vi "2108cdc.vi"() -> ()   [LabVIEW 2019]
doc: "This example performs writes and reads on a serial port, as directed by the user. You can press the Write and Read buttons, and change the Read Count, while the example is running.\n\nThe parameters set for the serial port must match the parameters of the connected instrument or device. In this example, the Read Count parameter specifies the number of bytes that the serial port reads. If there were more bytes at the port than the specified number, those bytes would not be read. If there were less bytes at the port than the specified number, you would receive a timeout error.\n\nThis example expands upon the flow control options for XON and XOFF, allowing the user to choose those control characters. Also, the user can enable or disable a termination character. Some devices require a termination character in order to identify the end of command strings. Some devices send a termination character to signify the end of data to be read. This example shows how you can end the Read operation once a termination character is detected in the buffer and/or append a termination character at the end of the Write data."
uses:
  <vilib>/Instr/_visa.llb/VISA Configure Serial Port (Instr).vi
panel:
  in  "Command List":string="stop\neol 1\nencode 1\nslist 0 0\nslist 1 1\nsrate 6000\ndec 500\ndeca 3\nnop\nstart\n"
  in  "Stop":bool
  out "Response":string=" 0.000, 0.000\n 0.000, 0.000\n 0.000, 0.000\n 0.000, 0.000\n 0.000, 0.000\n 0.000, 0.001\n 0.000, 0.001\n 0.000, 0.001\n 0.000, 0.001\n 0.000, 0.001\n 0.000, 0.000\n 0.000, 0.000\n 0.000, 0.000\n 0.000, 0.000\n 0.000, 0.000\n 0.000, 0.001\n 0.000, 0.000\n 0.000, 0.000\n 0.000, 0.000\n 0.000, 0.000\n 0.000, 0.000\n 0.000, 0.001\n 0.000, 0.001\n 0.000, 0.001\n 0.000, 0.000\n 0.000, 0.000\n 0.000, 0.000\n 0.000, 0.000\n 0.000, 0.000\n 0.000, 0.000\n 0.000, 0.000\n 0.000, 0.000\n 0.000, 0.000\n 0.000, 0.000\n 0.000, 0.000\n 0.000, 0.000\n 0.000, 0.000\n 0.000, 0.001\n 0.000, 0.001\n 0.000, 0.000\n 0.000, 0.000\n 0.000, 0.000\n 0.000, 0.001\n 0.000, 0.000\n 0.000, 0.000\n 0.000, 0.001\n 0.000, 0.000\n 0.000, 0.000\n 0.000, 0.000\n 0.000, 0.000\n 0.000, 0.001\n 0.000, 0.000\n 0.000, 0.000\n 0.000, 0.001\n 0.000, 0.000\n 0.000, 0.000\n 0.000, 0.000\n 0.000, 0.000\n 0.000, 0.000\n 0.000, 0.001\n 0.000, 0.000\n 0.000, 0.000\n 0.000, 0.000\n 0.000, 0.000\n 0.000, 0.001\n 0.000, 0.000\n 0.000, 0.000\n 0.000, 0.000\n 0.000, 0.000\n 0.000, 0.000\n 0.000, 0.000\n 0.000, 0.000\n 0.000, 0.000\n 0.000, 0.000\n 0.000, 0.000\n 0.000, 0.000\n"
  in  "2108 CDC Virtual COM":refnum<visa-resource-name>="COM11"
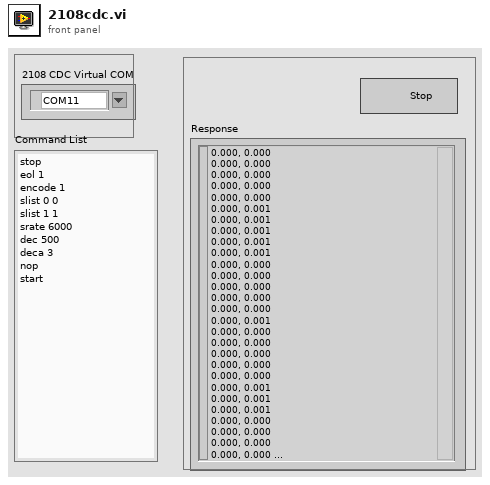
[diagram p1: front panel]
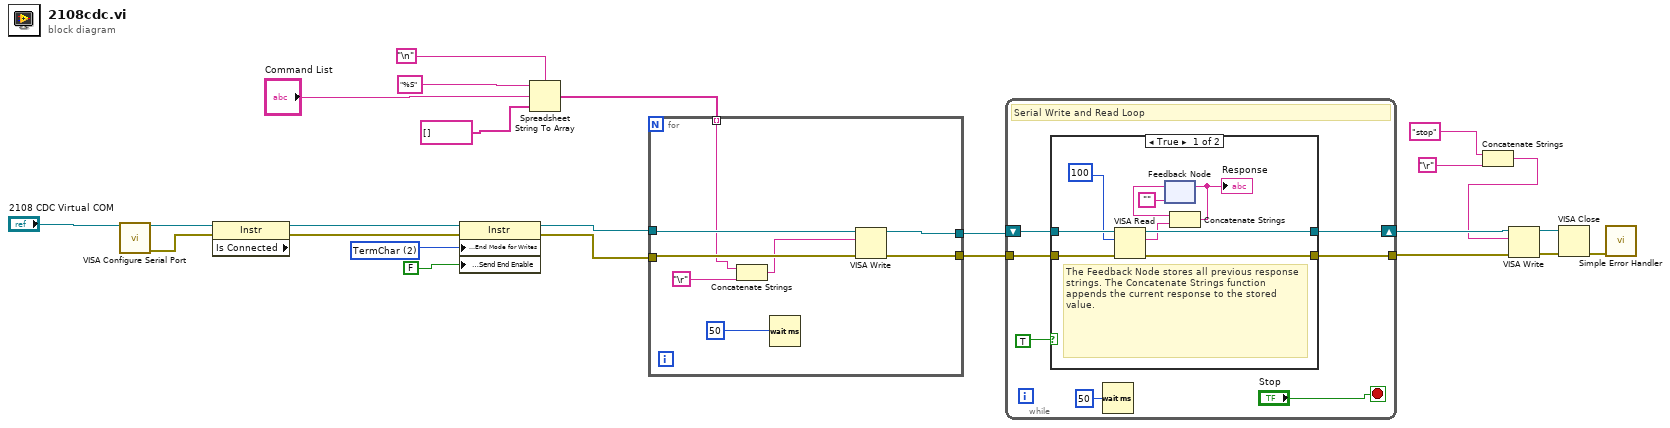
[diagram p0: block diagram]
diagram:
  w21 = u16 2 items=["None", "LastBit", "TermChar", "Break"] ("Serial Settings:Serial End Mode for Writes")
  n1 = call-poly "VISA Configure Serial Port"("VISA resource name"="2108 CDC Virtual COM") -> ("VISA resource name out"=w22:refnum<visa-resource-name>, "error out"=w24:errorcluster)  [unwired: 9 in, 4 out]
  n2 = property class="Instr" props=["Is Connected"](reference=w22, error in=w24) -> (reference out=w19:refnum<visa-resource-name>, error out=w18:errorcluster)  [unwired: 1 out]
  n3 = property class="Instr"(reference=w19, error in=w18, "Serial Settings:End Mode for Writes"=w21, "Message Based Settings:Send End Enable"=FALSE) -> (reference out=w1:refnum<visa-resource-name>, error out=w2:errorcluster)
  n4 = Spreadsheet String To Array(delimiter (Tab)="\n", format string="%S", spreadsheet string="Command List", array type (2D Dbl)=string[] []) -> (array=w14:string[])
  n5 = for {
    tunnel: w14 -> [w29] mode=indexing
    tunnel: w1 -> [w32]
    tunnel: w2 -> [w31]
    tunnel: [w26] -> w4
    tunnel: [w25] -> w3
    n6 = Concatenate Strings(w29, "\r") -> (w27:string)
    n7 = Wait (ms)(milliseconds to wait=u32 50) -> ()  [unwired: 1 out]
    n8 = VISA Write(VISA resource name=w32, write buffer=w27, error in (no error)=w31) -> (VISA resource name out=w26:refnum<visa-resource-name>, error out=w25:errorcluster)  [unwired: 1 out]
  }
  n9 = while {
    shift-right: [w39] -> w11
    shift-left: w4 -> [w35]
    tunnel: w3 -> [w34]
    tunnel: [w37] -> w8
    stop <- "Stop" stop-if-true
    # "Serial Write and Read Loop"
    n10 = case shown="True" TRUE {
      tunnel: [w46 w50] -> w39
      tunnel: w35 -> [w48 w50]
      tunnel: w34 -> [w47 w49]
      tunnel: [w45 w49] -> w37
      frame True {
        # "The Feedback Node stores all previous response strings. The Concatenate Strings function appends the current response to the stored value."
        n11 = VISA Read(VISA resource name=w48, byte count=100, error in (no error)=w47) -> (VISA resource name out=w46:refnum<visa-resource-name>, read buffer=w44:string, error out=w45:errorcluster)  [unwired: 1 out]
        n12 = feedback #1("") -> (w43:string)
        n13 = Concatenate Strings(w43, w44) -> (w42:string)
        "Response" <- w42
        n14 = feedback-in #1(w42) -> ()
      }
      frame False {
      }
    }
    n15 = Wait (ms)(milliseconds to wait=u32 50) -> ()  [unwired: 1 out]
  }
  n16 = Concatenate Strings("stop", "\r") -> (w5:string)
  n17 = VISA Write(VISA resource name=w11, write buffer=w5, error in (no error)=w8) -> (VISA resource name out=w10:refnum<visa-resource-name>, error out=w9:errorcluster)  [unwired: 1 out]
  n18 = VISA Close(VISA resource name=w10, error in (no error)=w9) -> (error out=w23:errorcluster)
  n19 = call <vilib>:"Simple Error Handler.vi"("error in (no error)"=w23) -> ()  [unwired: 1 in, 8 out]
